vi "Gen Freq.vi"(11 "Ref":waveform(dbl)={"t0"=timestamp(3571029165.757511 s since 1904-01-01), "dt"=1.9999999999999998e-05, "Y"=array[5000 elements]}) -> (3 "Ref_PLL_Out":waveform(dbl)={"t0"=timestamp(4.699999999999999 s since 1904-01-01), "dt"=1.9999999999999998e-05, "Y"=array[5000 elements]})   [LabVIEW 2020]
doc: "This VI adjusts both frequency and phase of one of the signals to be synchronized with the second one."
uses:
  <vilib>/measure/matone.llb/Extract Single Tone Information 1 Chan.vi
  <vilib>/measure/NI_MAPro.lvlib
  <vilib>/measure/NI_MABase.lvlib
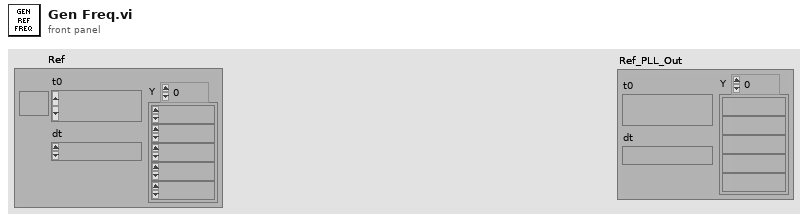
[diagram p1: front panel]
types:
  T1 = enum16{"Sine Wave", "Triangle Wave", "Square Wave", "Sawtooth Wave"}
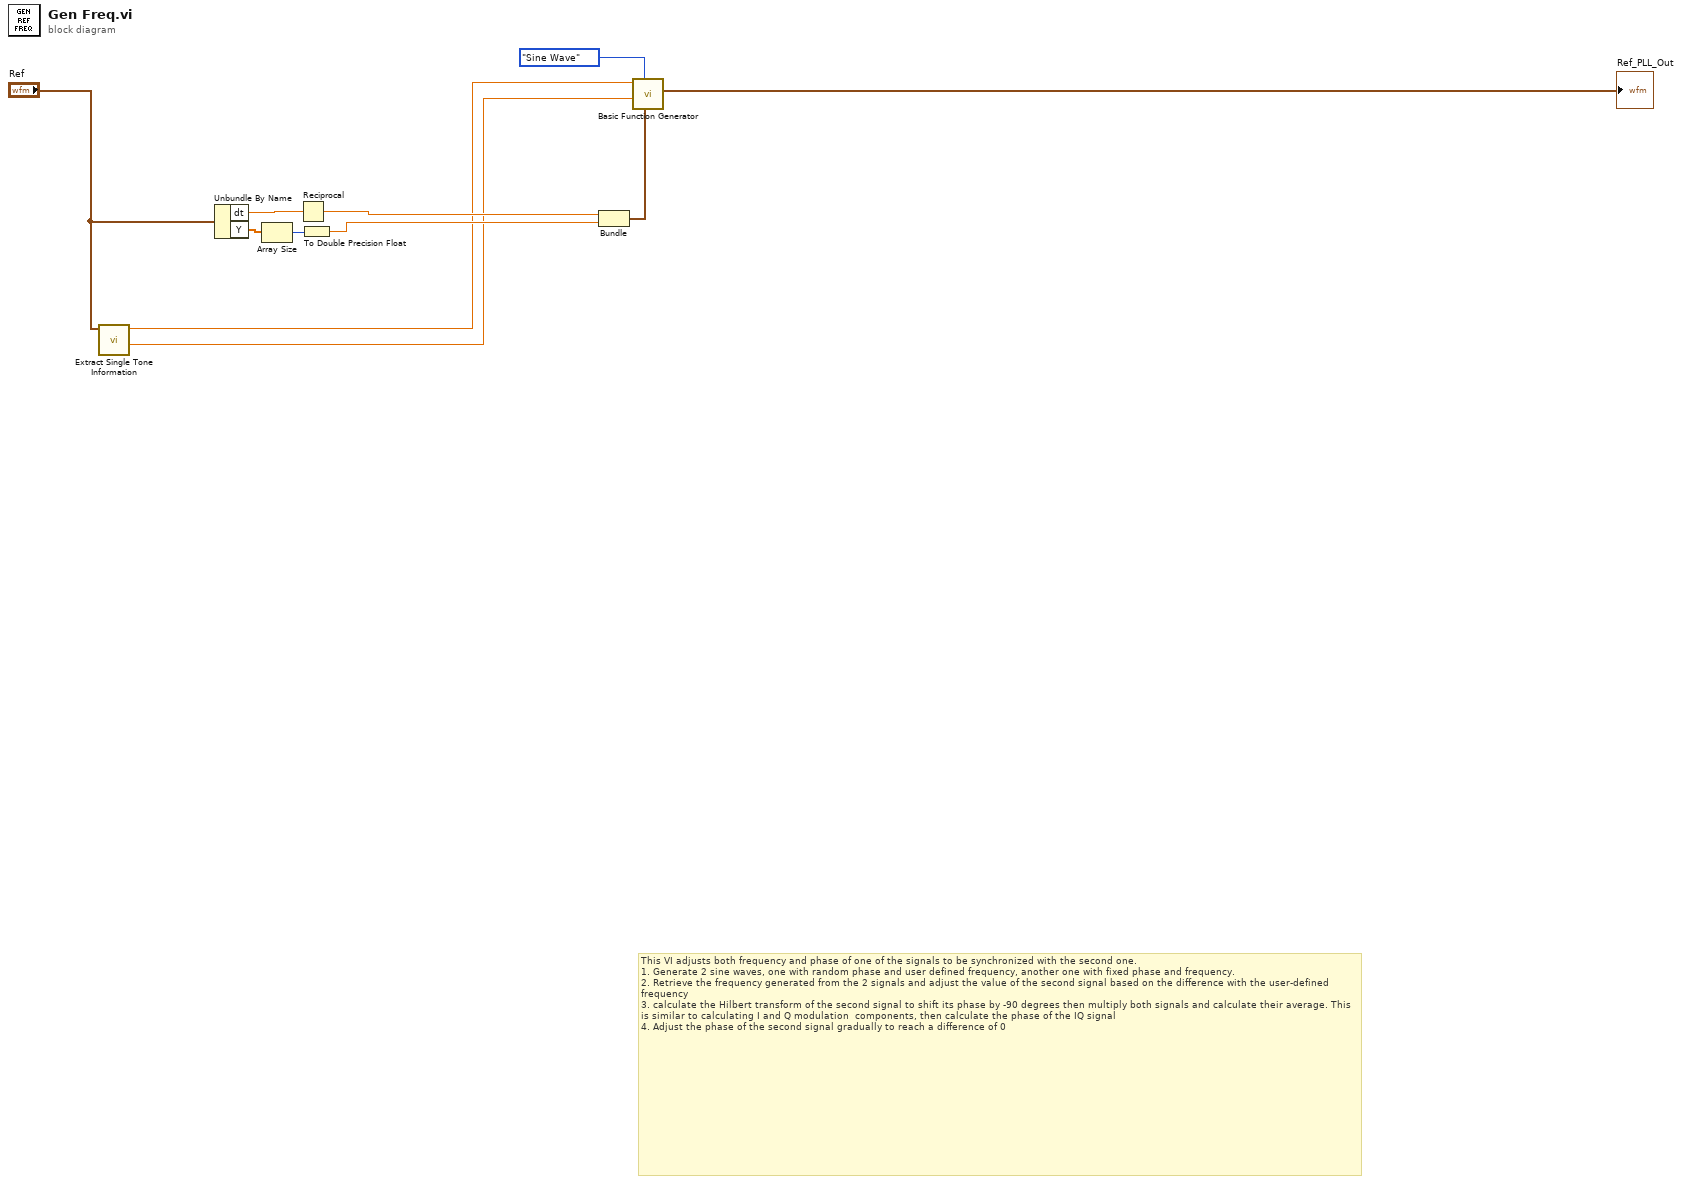
[diagram p0: block diagram]
diagram:
  # "This VI adjusts both frequency and phase of one of the signals to be synchronized with the second one.\n1. Generate 2 sine waves, one with random phase and user defined frequency, another one with fixed phase and frequency.\n2. Retrieve the frequency generated from the 2 signals and adjust the value of the second signal based on the difference with the user-defined frequency\n3. calculate the Hilbert transform of the second signal to shift its phase by -90 degrees then multiply both signals and calculate their average. This is similar to calculating I and Q modulation  components, then calculate the phase of the IQ signal\n4. Adjust the phase of the second signal gradually to reach a difference of 0"
  n1 = call-poly <vilib>:"Extract Single Tone Information.vi"("time signal in"="Ref") -> ("detected phase (deg)"=w4:dbl, "detected frequency"=w5:dbl)  [unwired: 5 in, 4 out]
  n2 = Unbundle By Name("Ref") -> ("dt"=w10:dbl, "Y"=w9:dbl[])
  n3 = Array Size(array=w9) -> (size(s)=w11:i32)
  n4 = Reciprocal(x=w10) -> (1/x=w8:dbl)
  n5 = To Double Precision Float(number=w11) -> (double precision float=w7:dbl)
  n6 = Bundle(w8, w7) -> (w2:cluster{dbl, dbl})  [unwired: 1 in]
  n7 = call <vilib>:"Basic Function Generator.vi"("sampling info"=w2, "signal type"=T1."Sine Wave", "phase"=w4, "frequency"=w5) -> ("signal out"=→"Ref_PLL_Out":waveform(dbl))  [unwired: 5 in, 2 out]
